vi "Measurement.IVCurve.UI.SetDependencies.vi"(8 "error in (no error)":errorcluster, 10 "Dependencies":T1, 11 "Measurement.IVCurve.UI in":refnum<class "Measurement.IVCurve.UI.lvclass">) -> (0 "error out":errorcluster, 3 "Measurement.IVCurve.UI out":refnum<class "Measurement.IVCurve.UI.lvclass">)   [LabVIEW 2017, in "Measurement.IVCurve.UI.lvclass"]
uses:
  Measurement.IVCurve.UI.lvclass
  Typedefs/Dependencies--Cluster.ctl
  Measurement.IVCurve/Measurement.IVCurve.lvclass
  Measurement.IVCurve.UI.lvclass/Measurement.IVCurve.UI.ctl
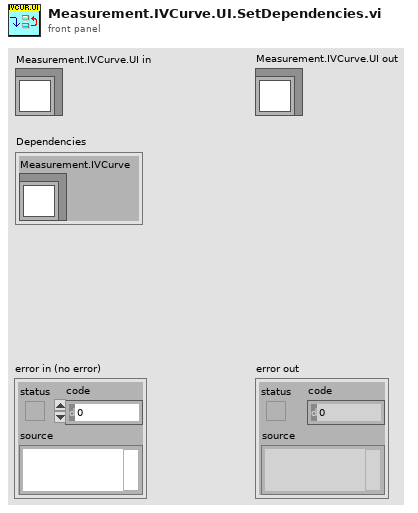
[diagram p1: front panel]
types:
  T1 = typedef "Measurement.IVCurve.UI.lvclass/Dependencies--Cluster.ctl" = cluster{"Measurement.IVCurve":refnum<class "Measurement.IVCurve.lvclass">}
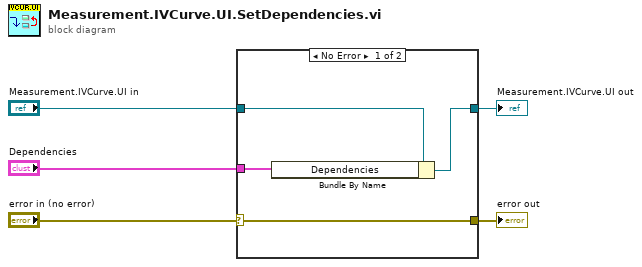
[diagram p0: block diagram]
diagram:
  n1 = case shown="No Error" "error in (no error)" {
    selector: "error in (no error)" -> [w9 w11]
    tunnel: [w9 w11] -> w4
    tunnel: [w6 w10] -> w2
    tunnel: "Measurement.IVCurve.UI in" -> [w8 w10]
    tunnel: "Dependencies" -> [w7 _]
    frame No Error {
      n2 = Bundle By Name(cluster=w8, "Dependencies"=w7) -> (w6:refnum<class "Measurement.IVCurve.UI.lvclass">)
    }
    frame Error {
    }
  }
  "error out" <- w4
  "Measurement.IVCurve.UI out" <- w2
